vi "Disconnection.vi"(8 "error in (no error)":errorcluster, 11 "PLC_Module in":refnum<class "PLC_Module.lvclass">) -> (0 "error out":errorcluster, 3 "PLC_Module out":refnum<class "PLC_Module.lvclass">)   [LabVIEW 2025, in "PLC_Module.lvlib" / "PLC_Module.lvclass"]
uses:
  PLC_Module.lvclass
  PLC_Module.lvclass/PLC_Module.ctl
  <vilib>/ActorFramework/Message Enqueuer/Message Enqueuer.lvclass/Message Enqueuer.ctl
  Write Connect.vi
  <vilib>/ActorFramework/Message Enqueuer/Enqueue.vi
  PLC_Abstr/PLC_Abstr Messages/Disconnection Msg/Disconnection Msg.lvclass
  C:/Program Files (x86)/National Instruments/LabVIEW 2025/vi.lib/ActorFramework/Message/Message.lvclass
  <vilib>/ActorFramework/Message Priority Queue/Priority Enqueue.vi
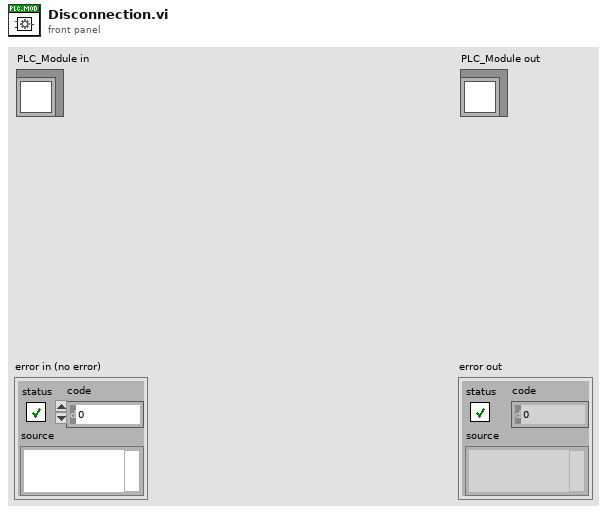
[diagram p1: front panel]
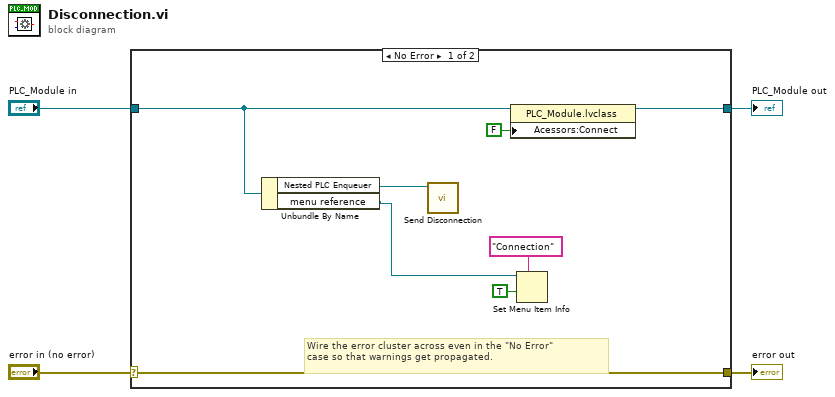
[diagram p0: block diagram]
diagram:
  n1 = case shown="No Error" "error in (no error)" {
    selector: "error in (no error)" -> [w12 w14]
    tunnel: [w12 w14] -> w3
    tunnel: [w9 w13] -> w1
    tunnel: "PLC_Module in" -> [w11 w13]
    frame No Error {
      # "Wire the error cluster across even in the \"No Error\"\ncase so that warnings get propagated."
      n2 = Unbundle By Name(w11) -> ("Nested PLC Enqueuer"=w10:refnum<class "Message Enqueuer.lvclass">, "menu reference"=w5:refnum<k9>)
      n3 = call "Send Disconnection.vi"("Message Enqueuer"=w10) -> ()  [unwired: 9 in, 2 out]
      n4 = property class="PLC_Module.lvclass"(reference=w11, "Acessors:Connect"=FALSE ("Connect")) -> (reference out=w9:refnum<class "PLC_Module.lvclass">)  [unwired: 1 in, 1 out]
      n5 = Set Menu Item Info(7:"Connection" ("item tag"), 9:TRUE ("enabled"), 11:w5) -> ()  [unwired: 4 in, 2 out]
    }
    frame Error {
    }
  }
  "error out" <- w3
  "PLC_Module out" <- w1
